vi "Data Access.vi"(8 "error in (no error)":errorcluster, 10 "Data Access Handler":refnum<class "Data Access Handler.lvclass">, 11 "DMM Immediate Measure Msg in":refnum<class "DMM Immediate Measure Msg.lvclass">) -> (0 "error out":errorcluster, 3 "DMM Immediate Measure Msg out":refnum<class "DMM Immediate Measure Msg.lvclass">)   [LabVIEW 2020, in "DMM Msg.lvlib" / "DMM Immediate Measure Msg.lvclass"]
doc: "Expose class private data to the front panel while letting the Data Access Handler class act on the data."
uses:
  DMM Immediate Measure Msg.lvclass
  C:/Current projects/WS/PPL/HDH.Actor Framework.Core.Msg.lvlibp/Flex Msg/Flex Msg.lvclass
  PPL/HDH.Actor Framework.Core.Msg.lvlibp/Flex Msg/Data Access Handlers/Data Access Handler/Data Access Handler.lvclass
  PPL/HDH.Actor Framework.Core.Publisher.lvlibp/Messages/Response Msg/Response Core/Controls/Ctl_SendFunction.ctl
  DMM Immediate Measure Msg.lvclass/DMM Immediate Measure Msg.ctl
  C:/Current projects/WS/PPL/HDH.Actor Framework.Core.Instrument Handler.lvlibp/Messages/Instrument Msg/Instrument Msg.lvclass
  PPL/HDH.Actor Framework.Core.Instrument Handler.lvlibp/Messages/Instrument Msg/Instrument Msg.lvclass
  PPL/HDH.Actor Framework.Core.Publisher.lvlibp
panel:
  in  "Publish?":bool=TRUE
  in  "Restore Range if Changed?":bool=TRUE
  in  "Max Time(ms)":i32=-1
  in  "Measurements to Acquire":i32=1
  in  "Message Priority":enum16{"Low", "Normal", "High"}(ring)=enum."Normal"
  in  "Timeout if Waiting":i32=-1
  in  "Send Function":T1=enum."Await Reply"
  in  "Cancel":bool
  in  "OK":bool
  # "Send details"
  # "Measure details"
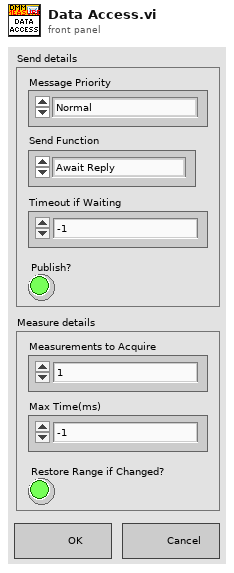
[diagram p1: front panel]
types:
  T1 = typedef "HDH.Actor Framework.Core.Publisher.lvlibp/Ctl_SendFunction.ctl" = enum16{"Send and Forget", "Request Reply", "Await Reply"}
  T2 = typedef "HDH.Actor Framework.Core.Actor.lvlibp/Message Enqueuer.lvclass/Message Priority.ctl" = enum16{"Low", "Normal", "High"}
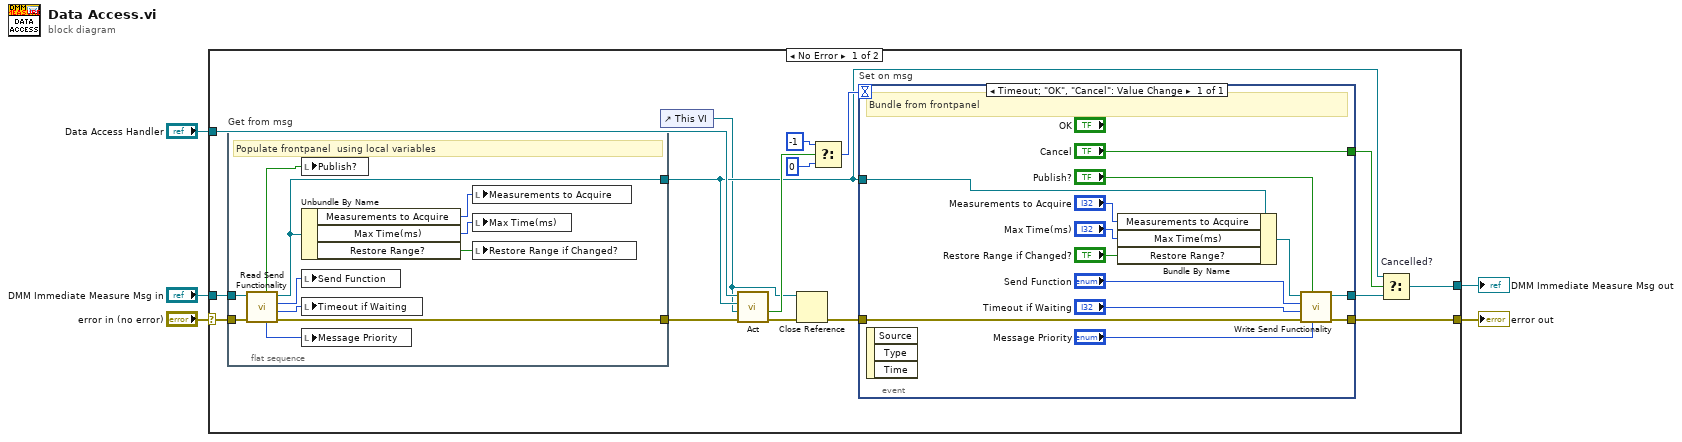
[diagram p0: block diagram]
diagram:
  n1 = case shown="No Error" "error in (no error)" {
    selector: "error in (no error)" -> [w21 w47]
    tunnel: [w14 w47] -> w4
    tunnel: [w9 w46] -> w2
    tunnel: "DMM Immediate Measure Msg in" -> [w12 w46]
    tunnel: "Data Access Handler" -> [w20 _]
    frame No Error {
      n2 = flat-sequence "Get from msg" {
        tunnel: w21 -> [w44]
        tunnel: [w42] -> w7
        tunnel: w12 -> [w45]
        tunnel: [w43] -> w19
        frame #0 {
          # "Populate frontpanel  using local variables"
          n3 = call "Read Send Functionality.vi"("error in (no error)"=w44, "Instrument Msg in"=w45) -> ("error out"=w43:errorcluster, "Timeout if Waiting"=w40:i32, "Send Function"=w41:T1, "Instrument Msg out"=w42:refnum<class "DMM Immediate Measure Msg.lvclass">, "Message Priority"=w39:T2, "Publish Data?"=w35:bool)  [unwired: 4 in]
          n4 = local write "Publish?"(w35) -> ()
          n5 = Unbundle By Name(w42) -> ("Measurements to Acquire"=w38:i32, "Max Time(ms)"=w37:i32, "Restore Range?"=w36:bool)
          n6 = local write "Send Function"(w41) -> ()
          n7 = local write "Timeout if Waiting"(w40) -> ()
          n8 = local write "Message Priority"(w39) -> ()
          n9 = local write "Measurements to Acquire"(w38) -> ()
          n10 = local write "Max Time(ms)"(w37) -> ()
          n11 = local write "Restore Range if Changed?"(w36) -> ()
        }
      }
      n12 = control-ref of="This VI"() -> (w6:refnum<vi>)
      n13 = call-dynamic "Act.vi"("error in (no error)"=w19, "VI Refnum in"=w6, "Flex Msg type"=w7, "Data Access Handler in"=w20) -> ("error out"=w11:errorcluster, "Await user action?"=w18:bool)  [unwired: 5 in, 1 out]
      n14 = Close Reference(reference=w6, error in (no error)=w11) -> (error out=w13:errorcluster)
      n15 = Select(t=-1, s=w18, f=0 ("t")) -> (s? t:f=w15:i32)
      n16 = event "Set on msg" shown="[0] Timeout;  \"OK\", \"Cancel\": Value Change" {
        selector: _ -> [_]
        dyn-events: _ -> [_]
        timeout: w15 -> [_]
        tunnel: [w29] -> w14
        tunnel: w13 -> [w30]
        tunnel: ["Cancel"] -> w10
        tunnel: [w32] -> w8
        tunnel: w7 -> [w33]
        event Timeout; "OK", "Cancel": Value Change {
          # "Bundle from frontpanel"
          n17 = event-data() -> ()  [unwired: 1 in, 3 out]
          n18 = Bundle By Name(cluster=w33, "Measurements to Acquire"="Measurements to Acquire", "Max Time(ms)"="Max Time(ms)", "Restore Range?"="Restore Range if Changed?") -> (w31:refnum<class "DMM Immediate Measure Msg.lvclass">)
          n19 = call "Write Send Functionality.vi"("Message Priority(Normal)"="Message Priority", "Publish Data?(T)"="Publish?", "error in (no error)"=w30, "Timeout if Waiting(-1ms)"="Timeout if Waiting", "Send Function(Await Reply)"="Send Function", "Instrument Msg in"=w31) -> ("error out"=w29:errorcluster, "Instrument Msg out"=w32:refnum<class "DMM Immediate Measure Msg.lvclass">)  [unwired: 4 in]
        }
      }
      n20 = Select "Cancelled?"(t=w7, s=w10, f=w8) -> (s? t:f=w9:refnum<class "DMM Immediate Measure Msg.lvclass">)
    }
    frame Error {
    }
  }
  "error out" <- w4
  "DMM Immediate Measure Msg out" <- w2
